vi "Events.vi"() -> ()   [LabVIEW 2026]
uses:
  SDL3/Events/MouseMotionEventData--cluster.ctl
  SDL3/Video/WindowID--integer.ctl
  SDL3/Mouse/MouseID--integer.ctl
  SDL3/Mouse/MouseButtonFlags--ring.ctl
  SDL3/Events/EventType--enum.ctl
  SDL3/Events/MouseButtonEventData--cluster.ctl
  SDL3/Events/MouseWheelEventData--cluster.ctl
  SDL3/Mouse/MouseWheelDirection--enum.ctl
  SDL3/Events/MouseDeviceEventData--cluster.ctl
  SDL3/Events/KeyboardDeviceEventData--cluster.ctl
  SDL3/Keyboard/KeyboardID--integer.ctl
  SDL3/Events/KeyboardEventData--cluster.ctl
  SDL3/Events/Scancode--integer.ctl
  SDL3/Keycode/Keycode--ring.ctl
  SDL3/Keycode/Keymod--ring.ctl
  SDL3/Events/QuitEventData--cluster.ctl
  SDL3/Video/WindowFlags--ring.ctl
  SDL3/Pixels/PixelFormat--enum.ctl
  SDL3/Render/TextureAccess-enum.ctl
  SDL3/Init/InitFlags--ring.ctl
  SDL3/Error/GetError-UiThread.vi
  SDL3/Pixels/PixelFormatEnumToU32.vi
  <vilib>/Utility/error.llb/Error Cluster From Error Code.vi
  SDL3/Init/Init.lvlib
  SDL3/Video/Video.lvlib
  SDL3/Render/Render.lvlib
  SDL3/Timer/Timer.lvlib
  SDL3/Events/Events.lvlib
  SDL3/Pixels/Pixels.lvlib
  SDL3/Mouse/Mouse.lvlib
  SDL3/Keyboard/Keyboard.lvlib
  SDL3/Keycode/Keycode.lvlib
panel:
  out "QuitEvent":T1
  out "KeyboardEvent":T2 {"Mod" items=["SDL_KMOD_NONE"=0, "SDL_KMOD_LSHIFT"=1, "SDL_KMOD_RSHIFT"=2, "SDL_KMOD_LCTRL"=64, "SDL_KMOD_RCTRL"=128, "SDL_KMOD_LALT"=256, "SDL_KMOD_RALT"=512, "SDL_KMOD_LGUI"=1024, "SDL_KMOD_RGUI"=2048, "SDL_KMOD_NUM"=4096, "SDL_KMOD_CAPS"=8192, "SDL_KMOD_MODE"=16384, "SDL_KMOD_SCROLL"=32768, "SDL_KMOD_CTRL"=192, "SDL_KMOD_SHIFT"=3, "SDL_KMOD_ALT"=768, "SDL_KMOD_GUI"=3072]; "Key" items=["SDLK_SCANCODE_MASK"=1073741824, "SDLK_UNKNOWN"=0, "SDLK_RETURN"=13, "SDLK_ESCAPE"=27, "SDLK_BACKSPACE"=8, "SDLK_TAB"=9, "SDLK_SPACE"=32, "SDLK_EXCLAIM"=33, "SDLK_DBLAPOSTROPHE"=34, "SDLK_HASH"=35, "SDLK_DOLLAR"=36, "SDLK_PERCENT"=37, "SDLK_AMPERSAND"=38, "SDLK_APOSTROPHE"=39, "SDLK_LEFTPAREN"=40, "SDLK_RIGHTPAREN"=41, "SDLK_ASTERISK"=42, "SDLK_PLUS"=43, "SDLK_COMMA"=44, "SDLK_MINUS"=45, "SDLK_PERIOD"=46, "SDLK_SLASH"=47, "SDLK_0"=48, "SDLK_1"=49, "SDLK_2"=50, "SDLK_3"=51, "SDLK_4"=52, "SDLK_5"=53, "SDLK_6"=54, "SDLK_7"=55, "SDLK_8"=56, "SDLK_9"=57, "SDLK_COLON"=58, "SDLK_SEMICOLON"=59, "SDLK_LESS"=60, "SDLK_EQUALS"=61, "SDLK_GREATER"=62, "SDLK_QUESTION"=63, "SDLK_AT"=64, "SDLK_LEFTBRACKET"=91, "SDLK_BACKSLASH"=92, "SDLK_RIGHTBRACKET"=93, "SDLK_CARET"=94, "SDLK_UNDERSCORE"=95, "SDLK_GRAVE"=96, "SDLK_A"=97, "SDLK_B"=98, "SDLK_C"=99, "SDLK_D"=100, "SDLK_E"=101, "SDLK_F"=102, "SDLK_G"=103, "SDLK_H"=104, "SDLK_I"=105, "SDLK_J"=106, "SDLK_K"=107, "SDLK_L"=108, "SDLK_M"=109, "SDLK_N"=110, "SDLK_O"=111, "SDLK_P"=112, "SDLK_Q"=113, "SDLK_R"=114, "SDLK_S"=115, "SDLK_T"=116, "SDLK_U"=117, "SDLK_V"=118, "SDLK_W"=119, "SDLK_X"=120, "SDLK_Y"=121, "SDLK_Z"=122, "SDLK_LEFTBRACE"=123, "SDLK_PIPE"=124, "SDLK_RIGHTBRACE"=125, "SDLK_TILDE"=126, "SDLK_DELETE"=127, "SDLK_PLUSMINUS"=177, "SDLK_CAPSLOCK"=1073741881, "SDLK_F1"=1073741882, "SDLK_F2"=1073741883, "SDLK_F3"=1073741884, "SDLK_F4"=1073741885, "SDLK_F5"=1073741886, "SDLK_F6"=1073741887, "SDLK_F7"=1073741888, "SDLK_F8"=1073741889, "SDLK_F9"=1073741890, "SDLK_F10"=1073741891, "SDLK_F11"=1073741892, "SDLK_F12"=1073741893, "SDLK_PRINTSCREEN"=1073741894, "SDLK_SCROLLLOCK"=1073741895, "SDLK_PAUSE"=1073741896, "SDLK_INSERT"=1073741897, "SDLK_HOME"=1073741898, "SDLK_PAGEUP"=1073741899, "SDLK_END"=1073741901, "SDLK_PAGEDOWN"=1073741902, "SDLK_RIGHT"=1073741903, "SDLK_LEFT"=1073741904, "SDLK_DOWN"=1073741905, "SDLK_UP"=1073741906, "SDLK_NUMLOCKCLEAR"=1073741907, "SDLK_KP_DIVIDE"=1073741908, "SDLK_KP_MULTIPLY"=1073741909, "SDLK_KP_MINUS"=1073741910, "SDLK_KP_PLUS"=1073741911, "SDLK_KP_ENTER"=1073741912, "SDLK_KP_1"=1073741913, "SDLK_KP_2"=1073741914, "SDLK_KP_3"=1073741915, "SDLK_KP_4"=1073741916, "SDLK_KP_5"=1073741917, "SDLK_KP_6"=1073741918, "SDLK_KP_7"=1073741919, "SDLK_KP_8"=1073741920, "SDLK_KP_9"=1073741921, "SDLK_KP_0"=1073741922, "SDLK_KP_PERIOD"=1073741923, "SDLK_APPLICATION"=1073741925, "SDLK_POWER"=1073741926, "SDLK_KP_EQUALS"=1073741927, "SDLK_F13"=1073741928, "SDLK_F14"=1073741929, "SDLK_F15"=1073741930, "SDLK_F16"=1073741931, "SDLK_F17"=1073741932, "SDLK_F18"=1073741933, "SDLK_F19"=1073741934, "SDLK_F20"=1073741935, "SDLK_F21"=1073741936, "SDLK_F22"=1073741937, "SDLK_F23"=1073741938, "SDLK_F24"=1073741939, "SDLK_EXECUTE"=1073741940, "SDLK_HELP"=1073741941, "SDLK_MENU"=1073741942, "SDLK_SELECT"=1073741943, "SDLK_STOP"=1073741944, "SDLK_AGAIN"=1073741945, "SDLK_UNDO"=1073741946, "SDLK_CUT"=1073741947, "SDLK_COPY"=1073741948, "SDLK_PASTE"=1073741949, "SDLK_FIND"=1073741950, "SDLK_MUTE"=1073741951, "SDLK_VOLUMEUP"=1073741952, "SDLK_VOLUMEDOWN"=1073741953, "SDLK_KP_COMMA"=1073741957, "SDLK_KP_EQUALSAS400"=1073741958, "SDLK_ALTERASE"=1073741977, "SDLK_SYSREQ"=1073741978, "SDLK_CANCEL"=1073741979, "SDLK_CLEAR"=1073741980, "SDLK_PRIOR"=1073741981, "SDLK_RETURN2"=1073741982, "SDLK_SEPARATOR"=1073741983, "SDLK_OUT"=1073741984, "SDLK_OPER"=1073741985, "SDLK_CLEARAGAIN"=1073741986, "SDLK_CRSEL"=1073741987, "SDLK_EXSEL"=1073741988, "SDLK_KP_00"=1073742000, "SDLK_KP_000"=1073742001, "SDLK_THOUSANDSSEPARATOR"=1073742002, "SDLK_DECIMALSEPARATOR"=1073742003, "SDLK_CURRENCYUNIT"=1073742004, "SDLK_CURRENCYSUBUNIT"=1073742005, "SDLK_KP_LEFTPAREN"=1073742006, "SDLK_KP_RIGHTPAREN"=1073742007, "SDLK_KP_LEFTBRACE"=1073742008, "SDLK_KP_RIGHTBRACE"=1073742009, "SDLK_KP_TAB"=1073742010, "SDLK_KP_BACKSPACE"=1073742011, "SDLK_KP_A"=1073742012, "SDLK_KP_B"=1073742013, "SDLK_KP_C"=1073742014, "SDLK_KP_D"=1073742015, "SDLK_KP_E"=1073742016, "SDLK_KP_F"=1073742017, "SDLK_KP_XOR"=1073742018, "SDLK_KP_POWER"=1073742019, "SDLK_KP_PERCENT"=1073742020, "SDLK_KP_LESS"=1073742021, "SDLK_KP_GREATER"=1073742022, "SDLK_KP_AMPERSAND"=1073742023, "SDLK_KP_DBLAMPERSAND"=1073742024, "SDLK_KP_VERTICALBAR"=1073742025, "SDLK_KP_DBLVERTICALBAR"=1073742026, "SDLK_KP_COLON"=1073742027, "SDLK_KP_HASH"=1073742028, "SDLK_KP_SPACE"=1073742029, "SDLK_KP_AT"=1073742030, "SDLK_KP_EXCLAM"=1073742031, "SDLK_KP_MEMSTORE"=1073742032, "SDLK_KP_MEMRECALL"=1073742033, "SDLK_KP_MEMCLEAR"=1073742034, "SDLK_KP_MEMADD"=1073742035, "SDLK_KP_MEMSUBTRACT"=1073742036, "SDLK_KP_MEMMULTIPLY"=1073742037, "SDLK_KP_MEMDIVIDE"=1073742038, "SDLK_KP_PLUSMINUS"=1073742039, "SDLK_KP_CLEAR"=1073742040, "SDLK_KP_CLEARENTRY"=1073742041, "SDLK_KP_BINARY"=1073742042, "SDLK_KP_OCTAL"=1073742043, "SDLK_KP_DECIMAL"=1073742044, "SDLK_KP_HEXADECIMAL"=1073742045, "SDLK_LCTRL"=1073742048, "SDLK_LSHIFT"=1073742049, "SDLK_LALT"=1073742050, "SDLK_LGUI"=1073742051, "SDLK_RCTRL"=1073742052, "SDLK_RSHIFT"=1073742053, "SDLK_RALT"=1073742054, "SDLK_RGUI"=1073742055, "SDLK_MODE"=1073742081, "SDLK_SLEEP"=1073742082, "SDLK_WAKE"=1073742083, "SDLK_CHANNEL_INCREMENT"=1073742084, "SDLK_CHANNEL_DECREMENT"=1073742085, "SDLK_MEDIA_PLAY"=1073742086, "SDLK_MEDIA_PAUSE"=1073742087, "SDLK_MEDIA_RECORD"=1073742088, "SDLK_MEDIA_FAST_FORWARD"=1073742089, "SDLK_MEDIA_REWIND"=1073742090, "SDLK_MEDIA_NEXT_TRACK"=1073742091, "SDLK_MEDIA_PREVIOUS_TRACK"=1073742092, "SDLK_MEDIA_STOP"=1073742093, "SDLK_MEDIA_EJECT"=1073742094, "SDLK_MEDIA_PLAY_PAUSE"=1073742095, "SDLK_MEDIA_SELECT"=1073742096, "SDLK_AC_NEW"=1073742097, "SDLK_AC_OPEN"=1073742098, "SDLK_AC_CLOSE"=1073742099, "SDLK_AC_EXIT"=1073742100, "SDLK_AC_SAVE"=1073742101, "SDLK_AC_PRINT"=1073742102, "SDLK_AC_PROPERTIES"=1073742103, "SDLK_AC_SEARCH"=1073742104, "SDLK_AC_HOME"=1073742105, "SDLK_AC_BACK"=1073742106, "SDLK_AC_FORWARD"=1073742107, "SDLK_AC_STOP"=1073742108, "SDLK_AC_REFRESH"=1073742109, "SDLK_AC_BOOKMARKS"=1073742110, "SDLK_SOFTLEFT"=1073742111, "SDLK_SOFTRIGHT"=1073742112, "SDLK_CALL"=1073742113, "SDLK_ENDCALL"=1073742114]}
  out "KeyboardDeviceEvent":T8
  out "MouseDeviceEvent":T9
  out "MouseWheelEvent":T11
  out "MouseButtonEvent":T13
  out "EventType":T14=enum."SDL_EVENT_QUIT"
  out "MouseMotionEvent":T15 {"State" items=["SDL_BUTTON_LEFT"=1, "SDL_BUTTON_MIDDLE"=2, "SDL_BUTTON_RIGHT"=3, "SDL_BUTTON_X1"=4, "SDL_BUTTON_X2"=5]}
  # "MOUSE"
  # "KEYBOARD"
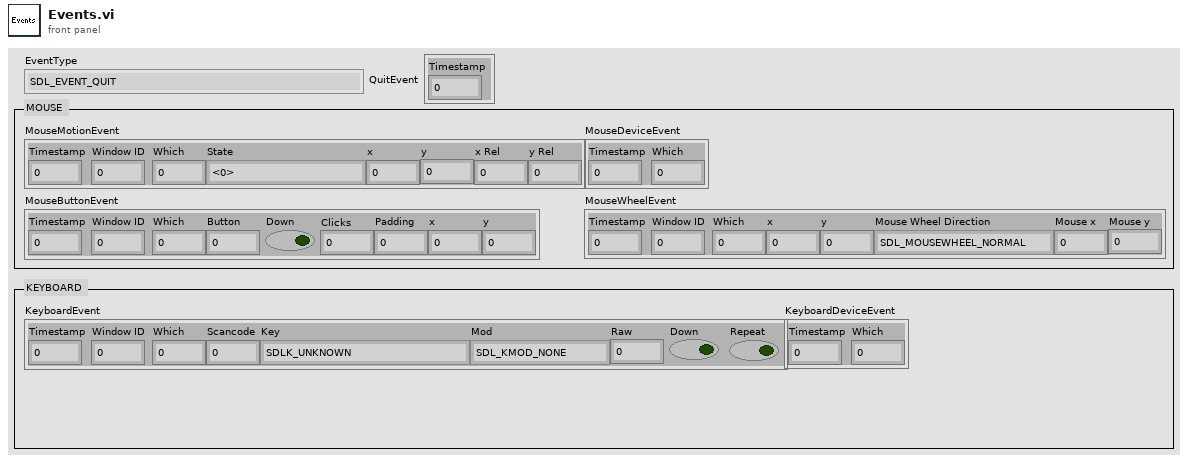
[diagram p1: front panel]
types:
  T1 = typedef "SDL3.lvlib/Events.lvlib/QuitEventData--cluster.ctl" = cluster{"Timestamp":u64}
  T2 = typedef "SDL3.lvlib/Events.lvlib/KeyboardEventData--cluster.ctl" = cluster{"Timestamp":u64, "Window ID":T3, "Which":T4, "Scancode":T5, "Key":T6, "Mod":T7, "Raw":u16, "Down":bool, "Repeat":bool}
  T3 = typedef "SDL3.lvlib/Video.lvlib/WindowID--integer.ctl" = u32
  T4 = typedef "SDL3.lvlib/Keyboard.lvlib/KeyboardID--integer.ctl" = u32
  T5 = typedef "SDL3.lvlib/Events.lvlib/Scancode--integer.ctl" = u32
  T6 = typedef "SDL3.lvlib/Keycode.lvlib/Keycode--ring.ctl" = u32
  T7 = typedef "SDL3.lvlib/Keycode.lvlib/Keymod--ring.ctl" = u16
  T8 = typedef "SDL3.lvlib/Events.lvlib/KeyboardDeviceEventData--cluster.ctl" = cluster{"Timestamp":u64, "Which":T4}
  T9 = typedef "SDL3.lvlib/Events.lvlib/MouseDeviceEventData--cluster.ctl" = cluster{"Timestamp":u64, "Which":T10}
  T10 = typedef "SDL3.lvlib/Mouse.lvlib/MouseID--integer.ctl" = u32
  T11 = typedef "SDL3.lvlib/Events.lvlib/MouseWheelEventData--cluster.ctl" = cluster{"Timestamp":u64, "Window ID":T3, "Which":T10, "x":sgl, "y":sgl, "Mouse Wheel Direction":T12, "Mouse x":sgl, "Mouse y":sgl}
  T12 = typedef "SDL3.lvlib/Mouse.lvlib/MouseWheelDirection--enum.ctl" = enum32{"SDL_MOUSEWHEEL_NORMAL", "SDL_MOUSEWHEEL_FLIPPED"}
  T13 = typedef "SDL3.lvlib/Events.lvlib/MouseButtonEventData--cluster.ctl" = cluster{"Timestamp":u64, "Window ID":T3, "Which":T10, "Button":u8, "Down":bool, "Clicks":u8, "Padding":u8, "x":sgl, "y":sgl}
  T14 = typedef "SDL3.lvlib/Events.lvlib/EventType--enum.ctl" = enum16{"LV_NONE", "LV_UNSUPPORTED", "SDL_EVENT_QUIT", "SDL_EVENT_LOCALE_CHANGED", "SDL_EVENT_SYSTEM_THEME_CHANGED", "SDL_EVENT_DISPLAY_ORIENTATION", "SDL_EVENT_DISPLAY_ADDED", "SDL_EVENT_DISPLAY_REMOVED", "SDL_EVENT_DISPLAY_MOVED", "SDL_EVENT_DISPLAY_DESKTOP_MODE_CHANGED", "SDL_EVENT_DISPLAY_CURRENT_MODE_CHANGED", "SDL_EVENT_DISPLAY_CONTENT_SCALE_CHANGED", "SDL_EVENT_WINDOW_SHOWN", "SDL_EVENT_WINDOW_HIDDEN", "SDL_EVENT_WINDOW_EXPOSED", "SDL_EVENT_WINDOW_MOVED", "SDL_EVENT_WINDOW_RESIZED", "SDL_EVENT_WINDOW_PIXEL_SIZE_CHANGED", "SDL_EVENT_WINDOW_METAL_VIEW_RESIZED", "SDL_EVENT_WINDOW_MINIMIZED", "SDL_EVENT_WINDOW_MAXIMIZED", "SDL_EVENT_WINDOW_RESTORED", "SDL_EVENT_WINDOW_MOUSE_ENTER", "SDL_EVENT_WINDOW_MOUSE_LEAVE", "SDL_EVENT_WINDOW_FOCUS_GAINED", "SDL_EVENT_WINDOW_FOCUS_LOST", "SDL_EVENT_WINDOW_CLOSE_REQUESTED", "SDL_EVENT_WINDOW_HIT_TEST", "SDL_EVENT_WINDOW_ICCPROF_CHANGED", "SDL_EVENT_WINDOW_DISPLAY_CHANGED", "SDL_EVENT_WINDOW_DISPLAY_SCALE_CHANGED", "SDL_EVENT_WINDOW_SAFE_AREA_CHANGED", "SDL_EVENT_WINDOW_OCCLUDED", "SDL_EVENT_WINDOW_ENTER_FULLSCREEN", "SDL_EVENT_WINDOW_LEAVE_FULLSCREEN", "SDL_EVENT_WINDOW_DESTROYED", "SDL_EVENT_WINDOW_HDR_STATE_CHANGED", "SDL_EVENT_KEY_DOWN", "SDL_EVENT_KEY_UP", "SDL_EVENT_TEXT_EDITING", "SDL_EVENT_TEXT_INPUT", "SDL_EVENT_KEYMAP_CHANGED", "SDL_EVENT_KEYBOARD_ADDED", "SDL_EVENT_KEYBOARD_REMOVED", "SDL_EVENT_TEXT_EDITING_CANDIDATES", "SDL_EVENT_MOUSE_MOTION", "SDL_EVENT_MOUSE_BUTTON_DOWN", "SDL_EVENT_MOUSE_BUTTON_UP", "SDL_EVENT_MOUSE_WHEEL", "SDL_EVENT_MOUSE_ADDED", "SDL_EVENT_MOUSE_REMOVED", "SDL_EVENT_JOYSTICK_AXIS_MOTION", "SDL_EVENT_JOYSTICK_BALL_MOTION", "SDL_EVENT_JOYSTICK_HAT_MOTION", "SDL_EVENT_JOYSTICK_BUTTON_DOWN", "SDL_EVENT_JOYSTICK_BUTTON_UP", "SDL_EVENT_JOYSTICK_ADDED", "SDL_EVENT_JOYSTICK_REMOVED", "SDL_EVENT_JOYSTICK_BATTERY_UPDATED", "SDL_EVENT_JOYSTICK_UPDATE_COMPLETE", "SDL_EVENT_GAMEPAD_AXIS_MOTION", "SDL_EVENT_GAMEPAD_BUTTON_DOWN", "SDL_EVENT_GAMEPAD_BUTTON_UP", "SDL_EVENT_GAMEPAD_ADDED", "SDL_EVENT_GAMEPAD_REMOVED", "SDL_EVENT_GAMEPAD_REMAPPED", "SDL_EVENT_GAMEPAD_TOUCHPAD_DOWN", "SDL_EVENT_GAMEPAD_TOUCHPAD_MOTION", "SDL_EVENT_GAMEPAD_TOUCHPAD_UP", "SDL_EVENT_GAMEPAD_SENSOR_UPDATE", "SDL_EVENT_GAMEPAD_UPDATE_COMPLETE", "SDL_EVENT_GAMEPAD_STEAM_HANDLE_UPDATED", "SDL_EVENT_FINGER_DOWN", "SDL_EVENT_FINGER_UP", "SDL_EVENT_FINGER_MOTION", "SDL_EVENT_CLIPBOARD_UPDATE", "SDL_EVENT_DROP_FILE", "SDL_EVENT_DROP_TEXT", "SDL_EVENT_DROP_BEGIN", "SDL_EVENT_DROP_COMPLETE", "SDL_EVENT_DROP_POSITION", "SDL_EVENT_AUDIO_DEVICE_ADDED", "SDL_EVENT_AUDIO_DEVICE_REMOVED", "SDL_EVENT_AUDIO_DEVICE_FORMAT_CHANGED", "SDL_EVENT_SENSOR_UPDATE", "SDL_EVENT_PEN_PROXIMITY_IN", "SDL_EVENT_PEN_PROXIMITY_OUT", "SDL_EVENT_PEN_DOWN", "SDL_EVENT_PEN_UP", "SDL_EVENT_PEN_BUTTON_DOWN", "SDL_EVENT_PEN_BUTTON_UP", "SDL_EVENT_PEN_MOTION", "SDL_EVENT_PEN_AXIS", "SDL_EVENT_CAMERA_DEVICE_ADDED", "SDL_EVENT_CAMERA_DEVICE_REMOVED", "SDL_EVENT_CAMERA_DEVICE_APPROVED", "SDL_EVENT_CAMERA_DEVICE_DENIED", "SDL_EVENT_RENDER_TARGETS_RESET", "SDL_EVENT_RENDER_DEVICE_RESET", "SDL_EVENT_POLL_SENTINEL", "SDL_EVENT_USER"}
  T15 = typedef "SDL3.lvlib/Events.lvlib/MouseMotionEventData--cluster.ctl" = cluster{"Timestamp":u64, "Window ID":T3, "Which":T10, "State":T16, "x":sgl, "y":sgl, "x Rel":sgl, "y Rel":sgl}
  T16 = typedef "SDL3.lvlib/Mouse.lvlib/MouseButtonFlags--ring.ctl" = u32
  T17 = typedef "SDL3.lvlib/Init.lvlib/InitFlags--ring.ctl" = u32
  T18 = typedef "SDL3.lvlib/Render.lvlib/TextureAccess-enum.ctl" = enum32{"SDL_TEXTUREACCESS_STATIC", "SDL_TEXTUREACCESS_STREAMING", "SDL_TEXTUREACCESS_TARGET"}
  T19 = typedef "SDL3.lvlib/Pixels.lvlib/PixelFormat--enum.ctl" = enum32{"SDL_PIXELFORMAT_UNKNOWN", "SDL_PIXELFORMAT_INDEX1LSB", "SDL_PIXELFORMAT_INDEX1MSB", "SDL_PIXELFORMAT_INDEX2LSB", "SDL_PIXELFORMAT_INDEX2MSB", "SDL_PIXELFORMAT_INDEX4LSB", "SDL_PIXELFORMAT_INDEX4MSB", "SDL_PIXELFORMAT_INDEX8", "SDL_PIXELFORMAT_RGB332", "SDL_PIXELFORMAT_XRGB4444", "SDL_PIXELFORMAT_XBGR4444", "SDL_PIXELFORMAT_XRGB1555", "SDL_PIXELFORMAT_XBGR1555", "SDL_PIXELFORMAT_ARGB4444", "SDL_PIXELFORMAT_RGBA4444", "SDL_PIXELFORMAT_ABGR4444", "SDL_PIXELFORMAT_BGRA4444", "SDL_PIXELFORMAT_ARGB1555", "SDL_PIXELFORMAT_RGBA5551", "SDL_PIXELFORMAT_ABGR1555", "SDL_PIXELFORMAT_BGRA5551", "SDL_PIXELFORMAT_RGB565", "SDL_PIXELFORMAT_BGR565", "SDL_PIXELFORMAT_RGB24", "SDL_PIXELFORMAT_BGR24", "SDL_PIXELFORMAT_XRGB8888", "SDL_PIXELFORMAT_RGBX8888", "SDL_PIXELFORMAT_XBGR8888", "SDL_PIXELFORMAT_BGRX8888", "SDL_PIXELFORMAT_ARGB8888", "SDL_PIXELFORMAT_RGBA8888", "SDL_PIXELFORMAT_ABGR8888", "SDL_PIXELFORMAT_BGRA8888", "SDL_PIXELFORMAT_XRGB2101010", "SDL_PIXELFORMAT_XBGR2101010", "SDL_PIXELFORMAT_ARGB2101010", "SDL_PIXELFORMAT_ABGR2101010", "SDL_PIXELFORMAT_RGB48", "SDL_PIXELFORMAT_BGR48", "SDL_PIXELFORMAT_RGBA64", "SDL_PIXELFORMAT_ARGB64", "SDL_PIXELFORMAT_BGRA64", "SDL_PIXELFORMAT_ABGR64", "SDL_PIXELFORMAT_RGB48_FLOAT", "SDL_PIXELFORMAT_BGR48_FLOAT", "SDL_PIXELFORMAT_RGBA64_FLOAT", "SDL_PIXELFORMAT_ARGB64_FLOAT", "SDL_PIXELFORMAT_BGRA64_FLOAT", "SDL_PIXELFORMAT_ABGR64_FLOAT", "SDL_PIXELFORMAT_RGB96_FLOAT", "SDL_PIXELFORMAT_BGR96_FLOAT", "SDL_PIXELFORMAT_RGBA128_FLOAT", "SDL_PIXELFORMAT_ARGB128_FLOAT", "SDL_PIXELFORMAT_BGRA128_FLOAT", "SDL_PIXELFORMAT_ABGR128_FLOAT", "SDL_PIXELFORMAT_YV12", "SDL_PIXELFORMAT_IYUV", "SDL_PIXELFORMAT_YUY2", "SDL_PIXELFORMAT_UYVY", "SDL_PIXELFORMAT_YVYU", "SDL_PIXELFORMAT_NV12", "SDL_PIXELFORMAT_NV21", "SDL_PIXELFORMAT_P010", "SDL_PIXELFORMAT_EXTERNAL_OES"}
  T20 = typedef "SDL3.lvlib/Video.lvlib/WindowFlags--ring.ctl" = u64
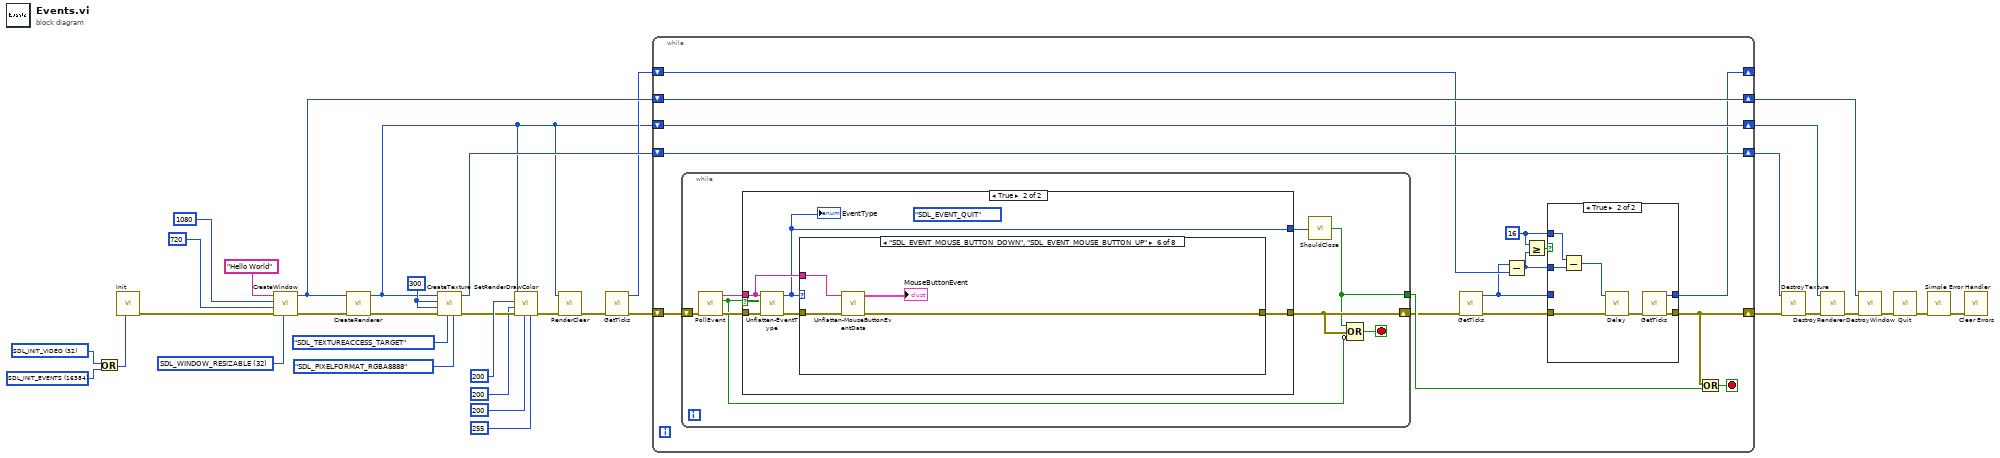
[diagram p0: block diagram]
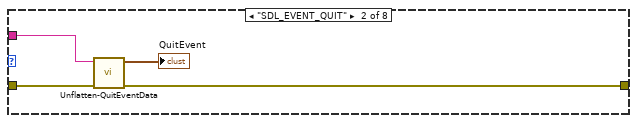
[diagram p4: hidden frame]
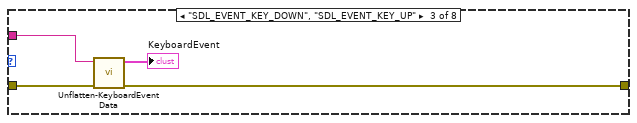
[diagram p5: hidden frame]
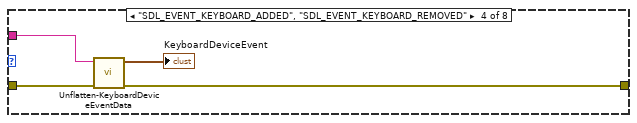
[diagram p6: hidden frame]
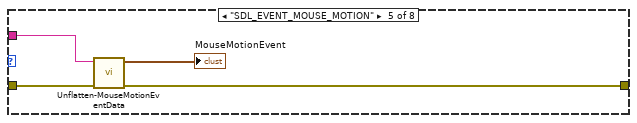
[diagram p7: hidden frame]
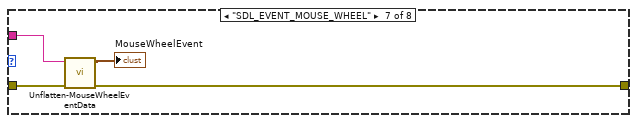
[diagram p8: hidden frame]
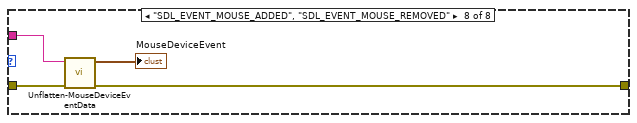
[diagram p9: hidden frame]
diagram:
  w9 = T17 16384 items=["NONE"=0, "SDL_INIT_AUDIO"=16, "SDL_INIT_VIDEO"=32, "SDL_INIT_JOYSTICK"=512, "SDL_INIT_HAPTIC"=4096, "SDL_INIT_GAMEPAD"=8192, "SDL_INIT_EVENTS"=16384, "SDL_INIT_SENSOR"=32768, "SDL_INIT_CAMER"=65536] ("y")
  w13 = T17 32 items=["NONE"=0, "SDL_INIT_AUDIO"=16, "SDL_INIT_VIDEO"=32, "SDL_INIT_JOYSTICK"=512, "SDL_INIT_HAPTIC"=4096, "SDL_INIT_GAMEPAD"=8192, "SDL_INIT_EVENTS"=16384, "SDL_INIT_SENSOR"=32768, "SDL_INIT_CAMER"=65536] ("InitFlags")
  w26 = 300 ("w")
  w31 = T20 32 items=["0"=0, "SDL_WINDOW_FULLSCREEN"=1, "SDL_WINDOW_OPENGL"=2, "SDL_WINDOW_OCCLUDED"=4, "SDL_WINDOW_HIDDEN"=8, "SDL_WINDOW_BORDERLESS"=16, "SDL_WINDOW_RESIZABLE"=32, "SDL_WINDOW_MINIMIZED"=64, "SDL_WINDOW_MAXIMIZED"=128, "SDL_WINDOW_MOUSE_GRABBED"=256, "SDL_WINDOW_INPUT_FOCUS"=512, "SDL_WINDOW_MOUSE_FOCUS"=1024, "SDL_WINDOW_EXTERNAL"=2048, "SDL_WINDOW_MODAL"=4096, "SDL_WINDOW_HIGH_PIXEL_DENSITY"=8192, "SDL_WINDOW_MOUSE_CAPTURE"=16384, "SDL_WINDOW_MOUSE_RELATIVE_MODE"=32768, "SDL_WINDOW_ALWAYS_ON_TOP"=65536, "SDL_WINDOW_UTILITY"=131072, "SDL_WINDOW_TOOLTIP"=262144, "SDL_WINDOW_POPUP_MENU"=524288, "SDL_WINDOW_KEYBOARD_GRABBED"=1048576, "SDL_WINDOW_VULKAN"=268435456, "SDL_WINDOW_METAL"=536870912, "SDL_WINDOW_TRANSPARENT"=1073741824, "SDL_WINDOW_NOT_FOCUSABLE"=2147483648] ("flags (0)")
  n1 = Or(x=w13, y=w9) -> (x .or. y?=w10:T17)
  n2 = call "Init.vi"("InitFlags"=w10) -> ("error out"=w34:errorcluster)  [unwired: 10 in]
  n3 = call "CreateWindow.vi"("Flags (0)"=w31, "No Error"=w34, "h"=720, "w"=1080, "Title"="Hello World" ("title")) -> ("Error Out"=w30:errorcluster, "Window [SDL_Window *]"=w22:i64)  [unwired: 5 in]
  n4 = call "CreateRenderer.vi"("No Error"=w30, "Window [SDL_Window *]"=w22) -> ("Error Out"=w27:errorcluster, "Renderer [SDL_Renderer *]"=w6:i64)  [unwired: 8 in]
  n5 = call "CreateTexture.vi"("Pixel Format"=PixelFormat--enum."SDL_PIXELFORMAT_RGBA8888" ("pixel_format"), "Texture Access"=TextureAccess-enum."SDL_TEXTUREACCESS_TARGET" ("texture_access"), "No Error"=w27, "h"=w26, "w"=w26, "Renderer [SDL_Renderer *]"=w6) -> ("error out"=w4:errorcluster, "Texture [SDL_Texture *]"=w21:i64)  [unwired: 4 in]
  n6 = call "SetRenderDrawColor.vi"("a"=u8 255, "b"=u8 200, "No Error"=w4, "g"=u8 200, "r"=u8 200, "Renderer [SDL_Renderer *]"=w6) -> ("error out"=w8:errorcluster)  [unwired: 5 in]
  n7 = call "RenderClear.vi"("No Error"=w8, "Renderer [SDL_Renderer *]"=w6) -> ("error out"=w7:errorcluster)  [unwired: 9 in]
  n8 = call "GetTicks.vi"("No Error"=w7) -> ("error out"=w12:errorcluster, "Ticks [ms]"=w11:u64)  [unwired: 9 in]
  n9 = while {
    shift-right: [w48] -> w18
    shift-left: w21 -> [w48]
    shift-right: [w47] -> w19
    shift-left: w6 -> [w47]
    shift-right: [w49] -> w20
    shift-left: w22 -> [w49]
    shift-right: [w35] -> w29
    shift-left: w12 -> [w39]
    shift-right: [w46] -> _
    shift-left: w11 -> [w44]
    stop <- w36 stop-if-true
    w43 = u64 16
    n10 = while {
      shift-right: [w52] -> w37
      shift-left: w39 -> [w57]
      tunnel: [w50] -> w38
      stop <- w56 stop-if-true
      n11 = call "PollEvent.vi"("No Error"=w57) -> ("error out"=w55:errorcluster, "Event Occured?"=w53:bool, "Event Binary Data"=w54:string)  [unwired: 8 in]
      n12 = case shown="True" w53 {
        tunnel: w55 -> [w58 w63]
        tunnel: w54 -> [_ w62]
        tunnel: [w58 w60] -> w52
        tunnel: [_ w59] -> w51
        frame False {
        }
        frame True {
          (unwired) EventType--enum."SDL_EVENT_QUIT" ("EventType")
          n13 = call "Unflatten-EventType.vi"("error in (no error)"=w63, "Event Binary Data In"=w62) -> ("error out"=w61:errorcluster, "EventType"=w59:T14)  [unwired: 8 in]
          "EventType" <- w59
          n14 = case shown="\"SDL_EVENT_MOUSE_BUTTON_DOWN\", \"SDL_EVENT_MOUSE_BUTTON_UP\"" w59 {
            tunnel: w62 -> [_ w67 w71 w75 w79 w83 w87 w91]
            tunnel: w61 -> [w64 w68 w72 w76 w80 w84 w88 w92]
            tunnel: [w64 w66 w70 w74 w78 w81 w86 w90] -> w60
            frame Default {
            }
            frame "SDL_EVENT_QUIT" {
              n15 = call "Unflatten-QuitEventData.vi"("error in (no error)"=w68, "Event Binary Data"=w67) -> ("error out"=w66:errorcluster, "Event Data"=→"QuitEvent":T1)  [unwired: 8 in]
            }
            frame "SDL_EVENT_KEY_DOWN", "SDL_EVENT_KEY_UP" {
              n16 = call "Unflatten-KeyboardEventData.vi"("error in (no error)"=w72, "Event Binary Data"=w71) -> ("error out"=w70:errorcluster, "Event Data"=→"KeyboardEvent":T2)  [unwired: 8 in]
            }
            frame "SDL_EVENT_KEYBOARD_ADDED", "SDL_EVENT_KEYBOARD_REMOVED" {
              n17 = call "Unflatten-KeyboardDeviceEventData.vi"("error in (no error)"=w76, "Event Binary Data"=w75) -> ("error out"=w74:errorcluster, "Event Data"=→"KeyboardDeviceEvent":T8)  [unwired: 8 in]
            }
            frame "SDL_EVENT_MOUSE_MOTION" {
              n18 = call "Unflatten-MouseMotionEventData.vi"("error in (no error)"=w80, "Event Binary Data"=w79) -> ("error out"=w78:errorcluster, "Event Data"=→"MouseMotionEvent":T15)  [unwired: 8 in]
            }
            frame "SDL_EVENT_MOUSE_BUTTON_DOWN", "SDL_EVENT_MOUSE_BUTTON_UP" {
              n19 = call "Unflatten-MouseButtonEventData.vi"("error in (no error)"=w84, "Event Binary Data"=w83) -> ("error out"=w81:errorcluster, "Event Data"=→"MouseButtonEvent":T13)  [unwired: 8 in]
            }
            frame "SDL_EVENT_MOUSE_WHEEL" {
              n20 = call "Unflatten-MouseWheelEventData.vi"("error in (no error)"=w88, "Event Binary Data"=w87) -> ("error out"=w86:errorcluster, "Event Data"=→"MouseWheelEvent":T11)  [unwired: 8 in]
            }
            frame "SDL_EVENT_MOUSE_ADDED", "SDL_EVENT_MOUSE_REMOVED" {
              n21 = call "Unflatten-MouseDeviceEventData.vi"("error in (no error)"=w92, "Event Binary Data"=w91) -> ("error out"=w90:errorcluster, "Event Data"=→"MouseDeviceEvent":T9)  [unwired: 8 in]
            }
          }
        }
      }
      n22 = call "ShouldClose.vi"("EventType"=w51) -> ("Close?"=w50:bool)
      n23 = Compound Arithmetic op=OR(w50, w52, invert w53) -> (w56:bool)
    }
    n24 = call "GetTicks.vi"("No Error"=w37) -> ("error out"=w45:errorcluster, "Ticks [ms]"=w40:u64)  [unwired: 9 in]
    n25 = Subtract(x=w40, y=w44) -> (x-y=w42:u64)
    n26 = Greater Or Equal?(x=w43, y=w42) -> (x >= y?=w41:bool)
    n27 = case shown="True" w41 {
      tunnel: [w93 w101] -> w35
      tunnel: [w94 w100] -> w46
      tunnel: w45 -> [w93 w99]
      tunnel: w43 -> [_ w98]
      tunnel: w42 -> [_ w97]
      tunnel: w40 -> [w94 _]
      frame False {
      }
      frame True {
        n28 = Subtract(x=w98, y=w97) -> (x-y=w95:u64)
        n29 = call "Delay.vi"("No Error"=w99, "ms"=w95) -> ("error out"=w96:errorcluster)  [unwired: 9 in]
        n30 = call "GetTicks.vi"("No Error"=w96) -> ("error out"=w101:errorcluster, "Ticks [ms]"=w100:u64)  [unwired: 9 in]
      }
    }
    n31 = Or(x=w35, y=w38) -> (x .or. y?=w36:bool)
  }
  n32 = call "DestroyTexture.vi"("No Error"=w29, "Texture [SDL_Texture *]"=w18) -> ("error out"=w23:errorcluster)  [unwired: 9 in]
  n33 = call "DestroyRenderer.vi"("No Error"=w23, "Rrenderer [SDL_Renderer *]"=w19) -> ("error out"=w28:errorcluster)  [unwired: 9 in]
  n34 = call "DestroyWindow.vi"("No Error"=w28, "Window [SDL_Window*]"=w20) -> ("Error Out"=w33:errorcluster)  [unwired: 9 in]
  n35 = call "Quit.vi"("No Error"=w33) -> ("error out"=w15:errorcluster)  [unwired: 10 in]
  n36 = call <vilib>:"Simple Error Handler.vi"("error in (no error)"=w15) -> ("error out"=w14:errorcluster)  [unwired: 4 in, 4 out]
  n37 = call <vilib>:"Clear Errors.vi"("error in (no error)"=w14) -> ()  [unwired: 5 in, 2 out]
